vi "Gen_Random_Sine.vi"(6 "sampling info for sine":cluster{"Fs":dbl, "#s":dbl}={"Fs"=10000.0, "#s"=2000.0}) -> (3 "data":sgl[](graph))   [LabVIEW 2020]
uses:
  <vilib>/measure/NI_MABase.lvlib
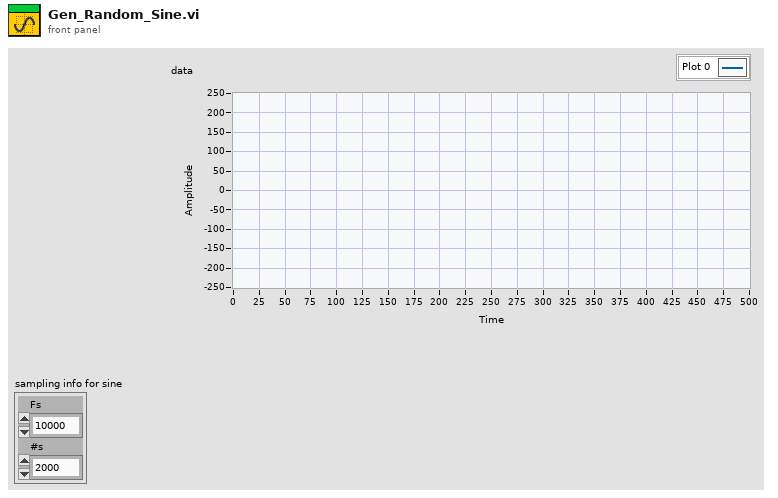
[diagram p1: front panel]
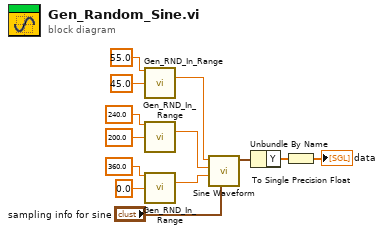
[diagram p0: block diagram]
diagram:
  n1 = call "Gen_RND_In_Range.vi"("Upper Bound"=55.0 ("frequency"), "Lower Bound"=45.0 ("Variation%")) -> ("RND_In_Range"=w10:dbl)  [unwired: 13 in]
  n2 = call "Gen_RND_In_Range.vi"("Upper Bound"=240.0 ("amplitude"), "Lower Bound"=200.0 ("variation")) -> ("RND_In_Range"=w8:dbl)  [unwired: 13 in]
  n3 = call "Gen_RND_In_Range.vi"("Upper Bound"=360.0 ("phase(digree)"), "Lower Bound"=0.0 ("Range")) -> ("RND_In_Range"=w13:dbl)  [unwired: 13 in]
  n4 = call <vilib>:"Sine Waveform.vi"("sampling info"="sampling info for sine", "phase"=w13, "amplitude"=w8, "frequency"=w10) -> ("signal out"=w12:waveform(dbl))  [unwired: 6 in, 1 out]
  n5 = Unbundle By Name(w12) -> ("Y"=w3:dbl[])
  n6 = To Single Precision Float(number=w3) -> (single precision float=→"data":sgl[])
